vi "SetupModel.vi"(8 "error in (no error)":errorcluster) -> (0 "error out":errorcluster, 3 "Model out":refnum<class "Model.lvclass">)   [LabVIEW 2016, in "Model.lvclass"]
uses:
  Model.lvclass
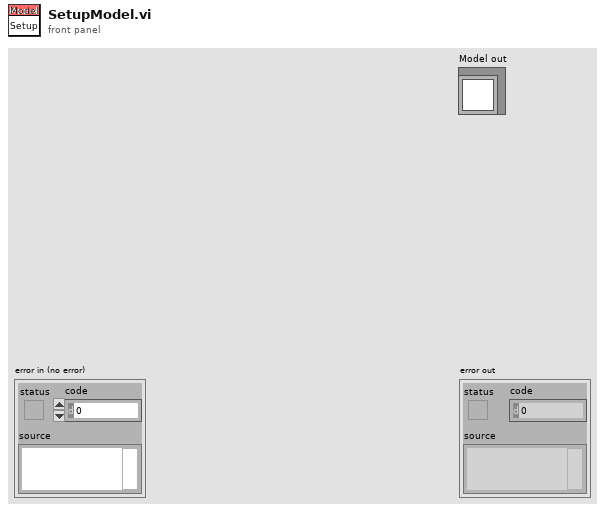
[diagram p1: front panel]
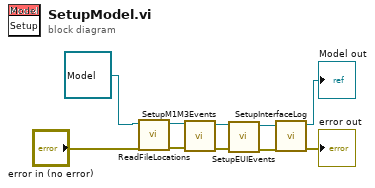
[diagram p0: block diagram]
diagram:
  n1 = call "ReadFileLocations.vi"("error in (no error)"="error in (no error)", "Model in"=refnum<class "Model.lvclass"> refnum ("Model.lvclass")) -> ("error out"=w1:errorcluster, "Model out"=w2:refnum<class "Model.lvclass">)  [unwired: 7 in, 1 out]
  n2 = call "SetupM1M3Events.vi"("error in (no error)"=w1, "Model in"=w2) -> ("error out"=w8:errorcluster, "Model out"=w6:refnum<class "Model.lvclass">)  [unwired: 8 in]
  n3 = call "SetupEUIEvents.vi"("error in (no error)"=w8, "Model in"=w6) -> ("error out"=w7:errorcluster, "Model out"=w5:refnum<class "Model.lvclass">)  [unwired: 8 in]
  n4 = call "SetupInterfaceLog.vi"("error in (no error)"=w7, "Model in"=w5) -> ("error out"=→"error out":errorcluster, "Model out"=→"Model out":refnum<class "Model.lvclass">)  [unwired: 8 in]
